vi "RIB Req - UDP Enable ROV A B TMS.vi"(0 "Limits File Path":path, 5 "Results File Path":path, 11 "error in":errorcluster) -> (4 "Results Data Array":string[][](array[string]), 15 "error out":errorcluster)   [LabVIEW 2024]
doc: "Template test"
uses:
  <vilib>/addons/_JKI Toolkits/State Machine/_JKI_lib_State_Machine.llb/Select State(s)_err__jki_lib_state_machine.vi
  <vilib>/addons/_JKI Toolkits/State Machine/_JKI_lib_State_Machine.llb/Select State(s)_bool__jki_lib_state_machine.vi
  <vilib>/addons/_JKI Toolkits/State Machine/_JKI_lib_State_Machine.llb/Periodic Trigger__ogtk__JKI-SM__jki_lib_state_machine.vi
  <userlib>/_OpenG.lib/file/file.llb/Strip Path Extension - String__ogtk.vi
  <vilib>/Utility/file.llb/Read Delimited Spreadsheet (string).vi
  <userlib>/_OpenG.lib/file/file.llb/openg_file.lvlib
  <userlib>/_OpenG.lib/appcontrol/appcontrol.llb/openg_application_control.lvlib
  <userlib>/_OpenG.lib/time/time.llb/openg_time.lvlib
  <vilib>/Utility/file.llb/Write Delimited Spreadsheet (string).vi
panel:
  in  "Connect":string
  in  "Connect Fail":string
  out "Timeout (Read States) 3":dbl(slide) scale=0.0..10.0
  out "Timeout (Read States)":dbl(slide) scale=0.0..15.0
  out "Timeout (Read States) 2":dbl(slide) scale=0.0..10.0
  out "ROV A Enabled":bool
  out "ROV B Enabled":bool
  out "TMS Enabled":bool
  in  "Read Normal Operation":string
  in  "Read Wait for Start":string
  in  "Read TMS":string
  in  "Read ROV B":string
  in  "Read ROV A":string
  out "Results Data 8":string[](array[string])
  out "Results Data 7":string[](array[string])
  out "Results Data 6":string[](array[string])
  in  "5A Test":bool
  in  "task out":refnum<k21>
  in  "UDP Read":string
  in  "connection ID":refnum<k16>
  in  "Exit":bool
  # "Enable ROV A, ROV B + TMS  Test"
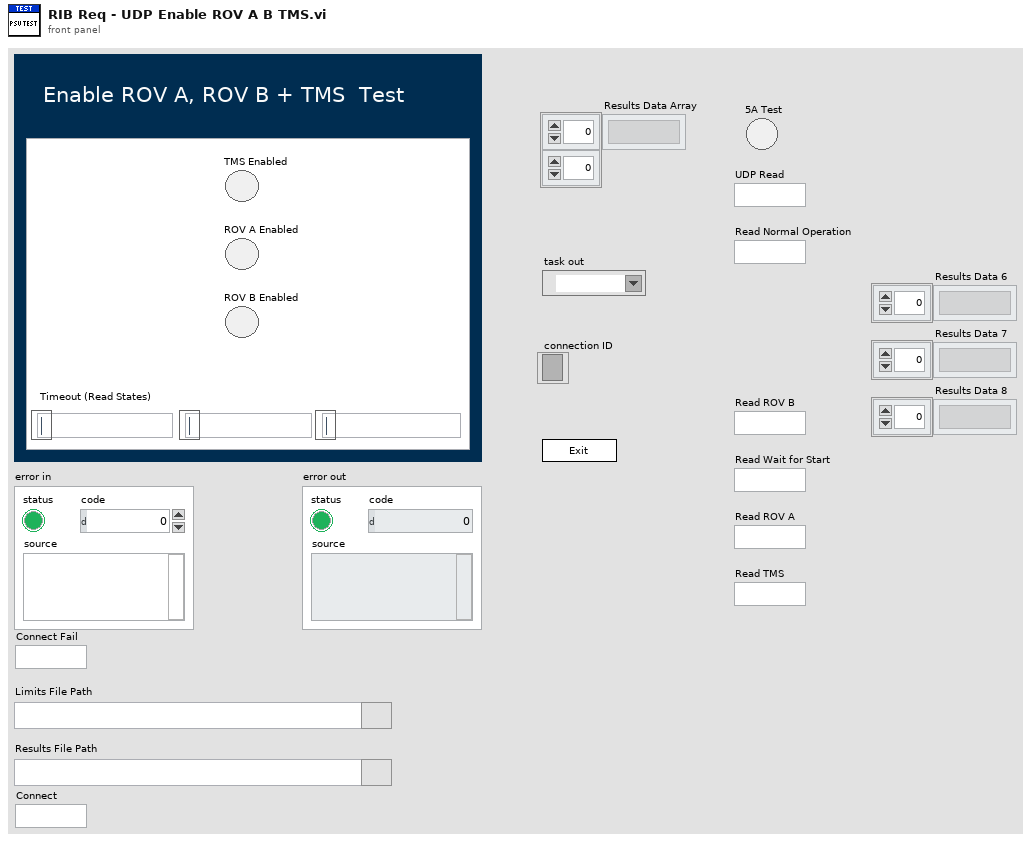
[diagram p1: front panel]
types:
  T1 = enum32{"Invalid", "Standard", "Closed", "Hidden", "Minimized", "Maximized"}
  T2 = enum32{"invalid app kind", "Development System", "Run Time System", "Student Edition", "Embedded LabVIEW", "Evaluation", "Custom"}
  T3 = typedef "FGV - Enum" = enum16{"Cleanup", "Get Data", "Open UDP", "Initialise DAQ", "Initialise I2C"}
  T4 = enum16{"Start Timer", "Get Time", "Pause", "Unpause"}
  T5 = cluster{"Core":cluster{"Current VI Reference":refnum<vi>, "Close Panel on Exit?":bool}, "Limits File Path":path, "Test Limits":string[][], "Results Data Array":string[][], "Results File Path":path, "UDP Read":string, "connection ID":refnum<k16>, "task out":refnum<k21>, "5A Test":bool, "Connect Fail":string, "Connect":string, "Read ROV A":string, "Read ROV B":string, "Read TMS":string, "Read Wait for Start":string, "Read Normal Operation":string}
  T6 = cluster{"Current VI Reference":refnum<vi>, "Close Panel on Exit?":bool}
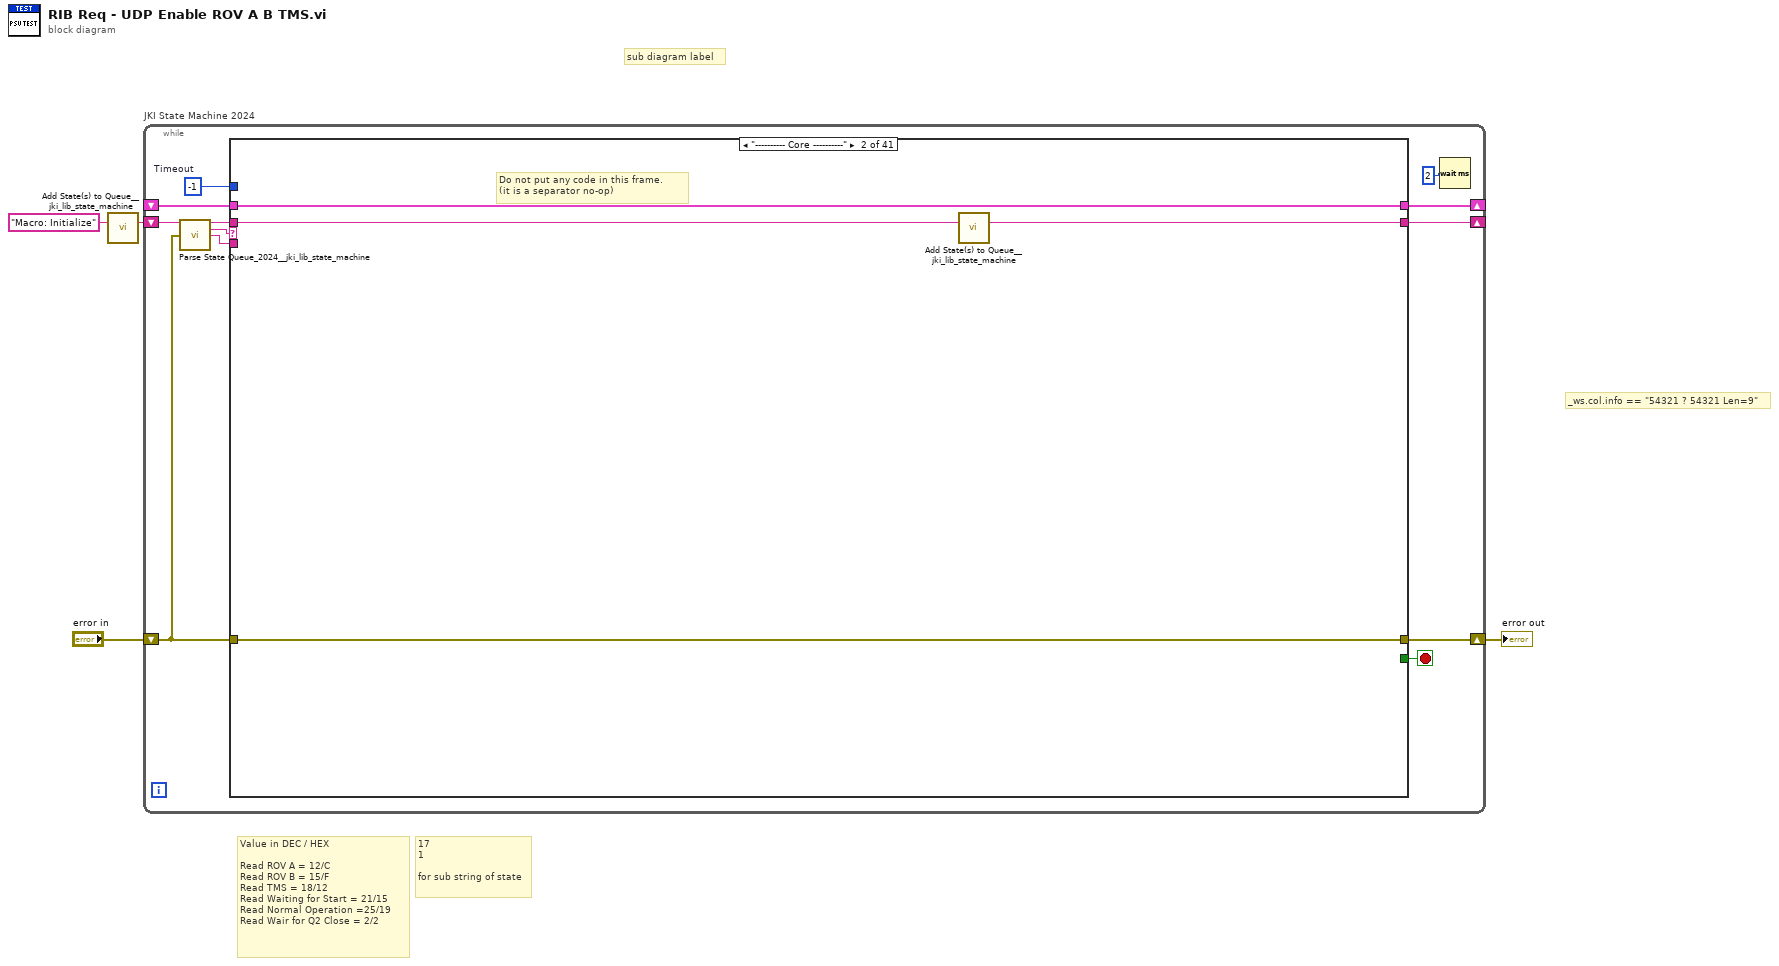
[diagram p0: block diagram]
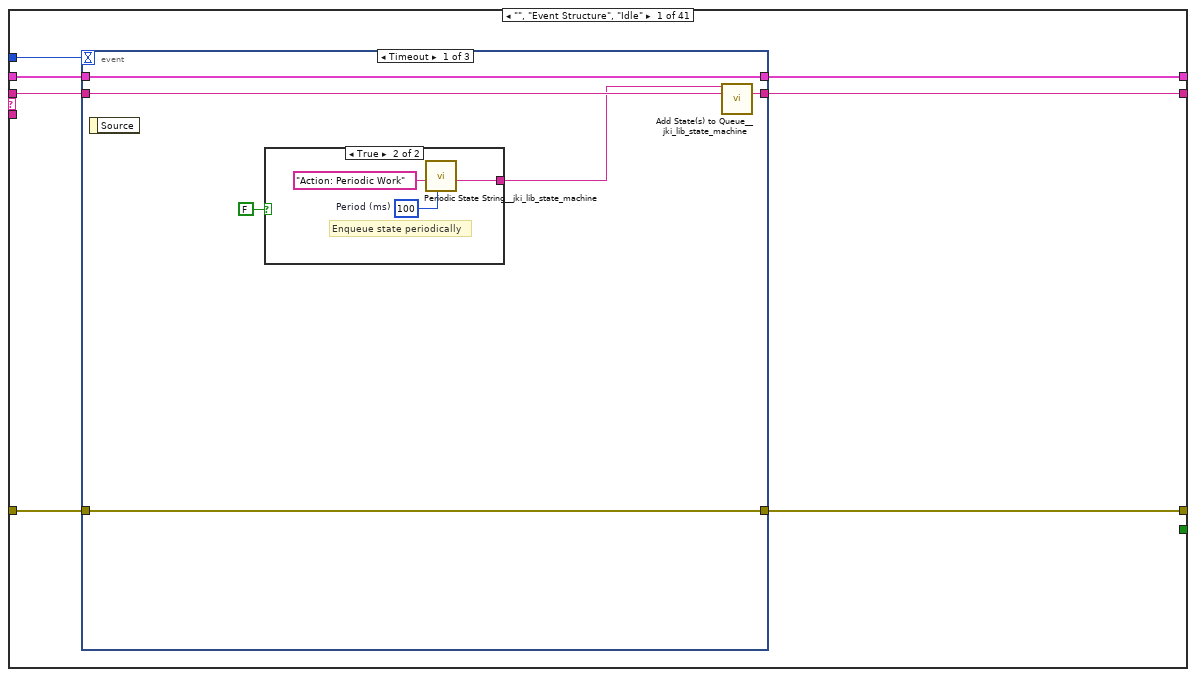
[diagram p2: hidden frame]
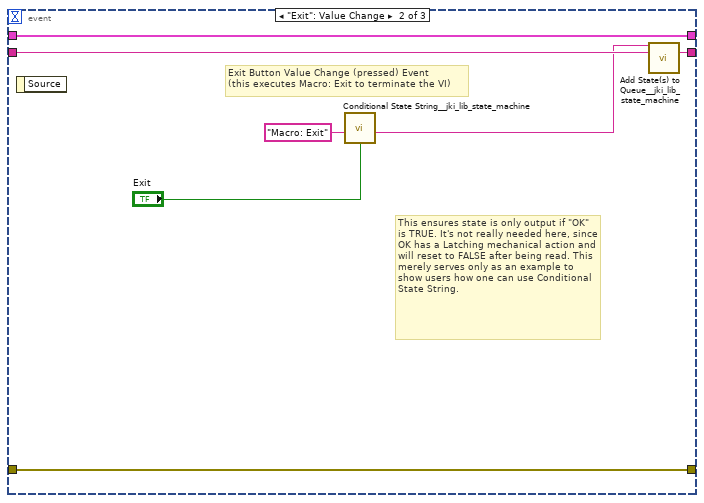
[diagram p4: hidden frame]
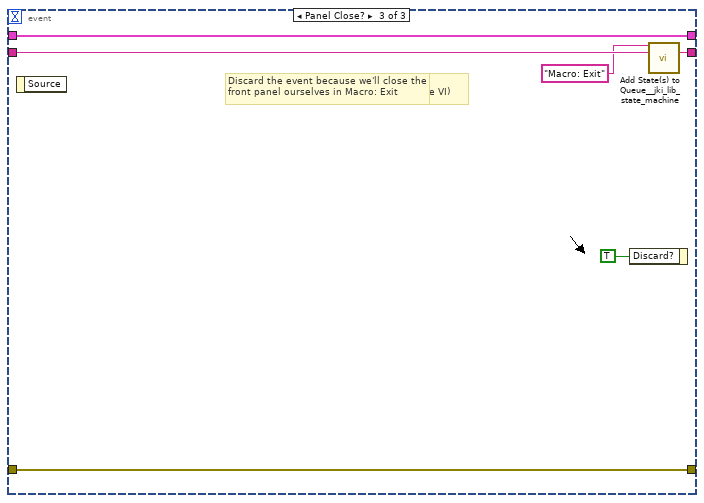
[diagram p5: hidden frame]
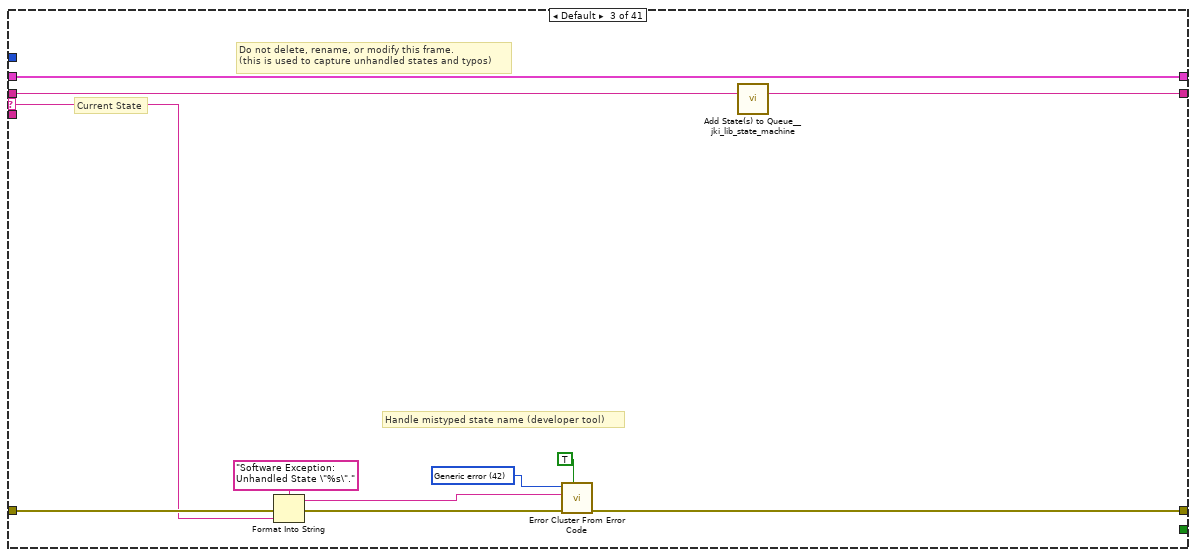
[diagram p6: hidden frame]
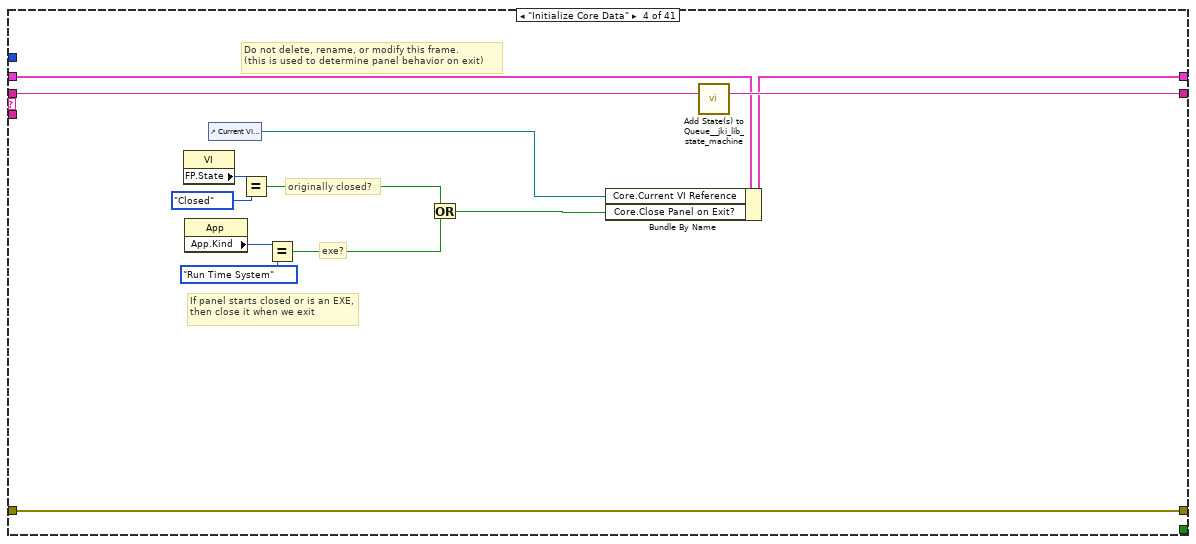
[diagram p7: hidden frame]
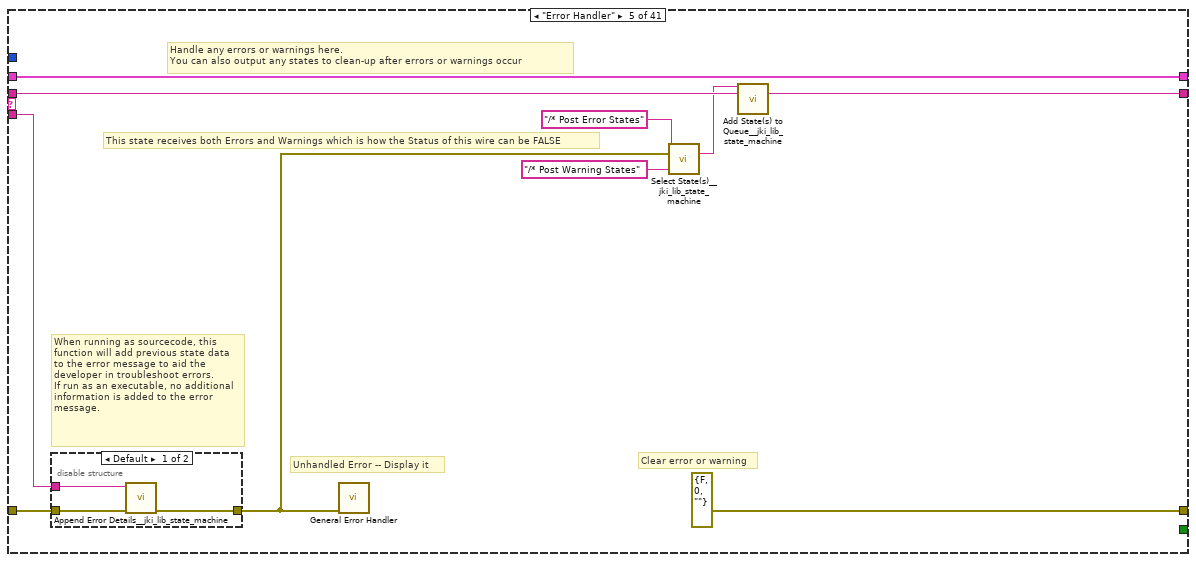
[diagram p8: hidden frame]
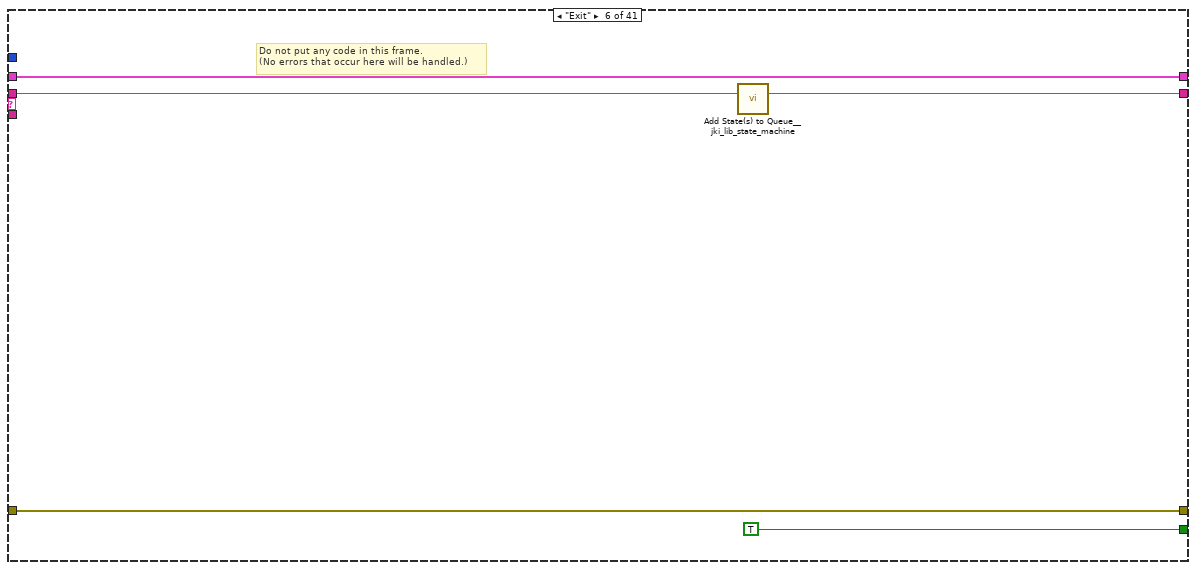
[diagram p10: hidden frame]
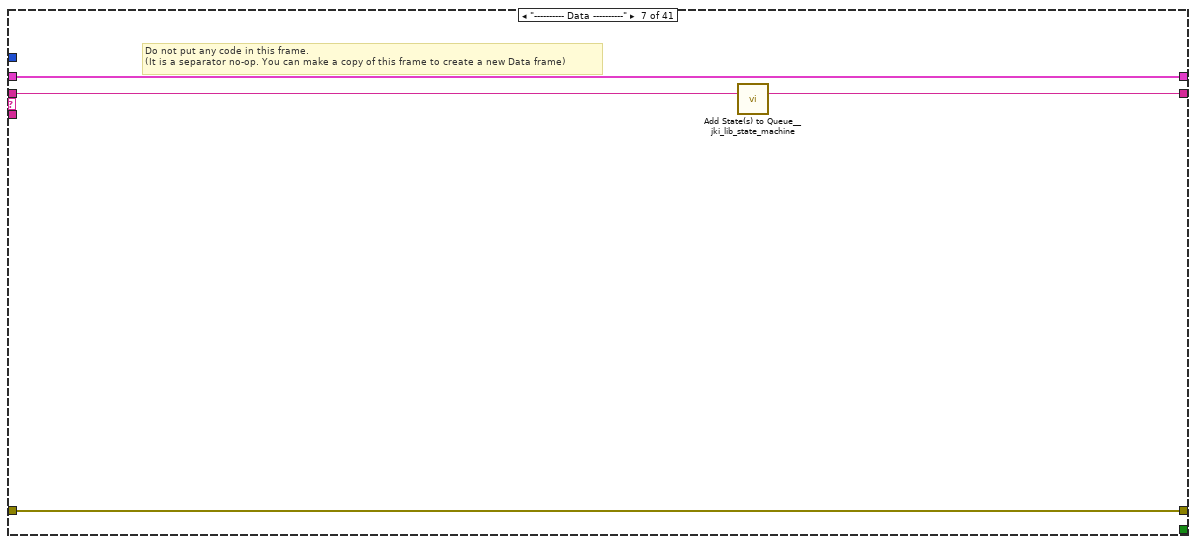
[diagram p11: hidden frame]
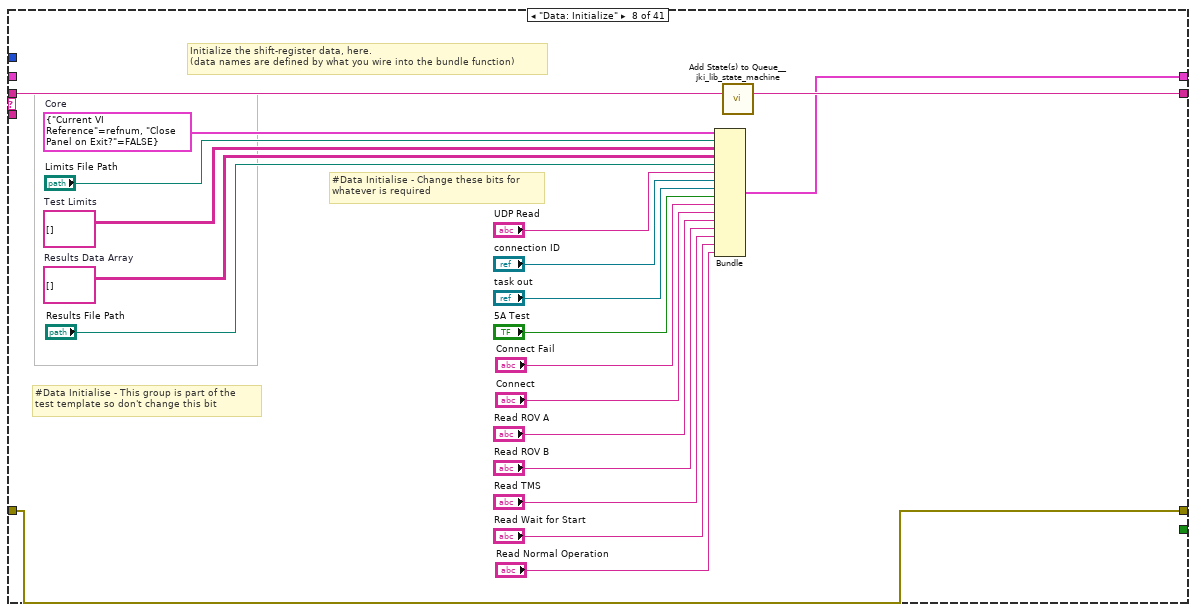
[diagram p12: hidden frame]
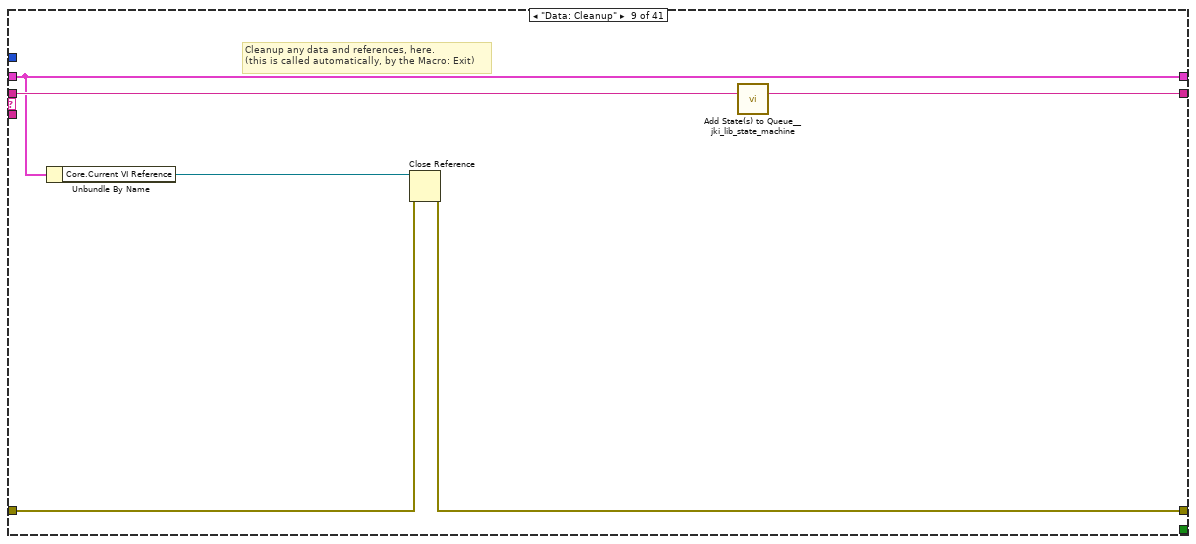
[diagram p13: hidden frame]
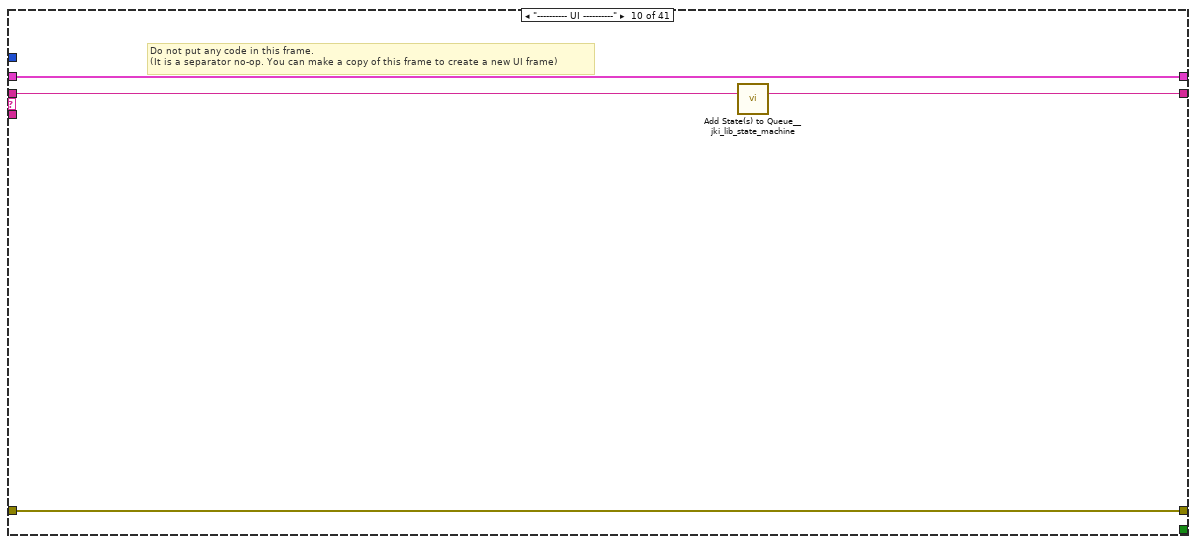
[diagram p14: hidden frame]
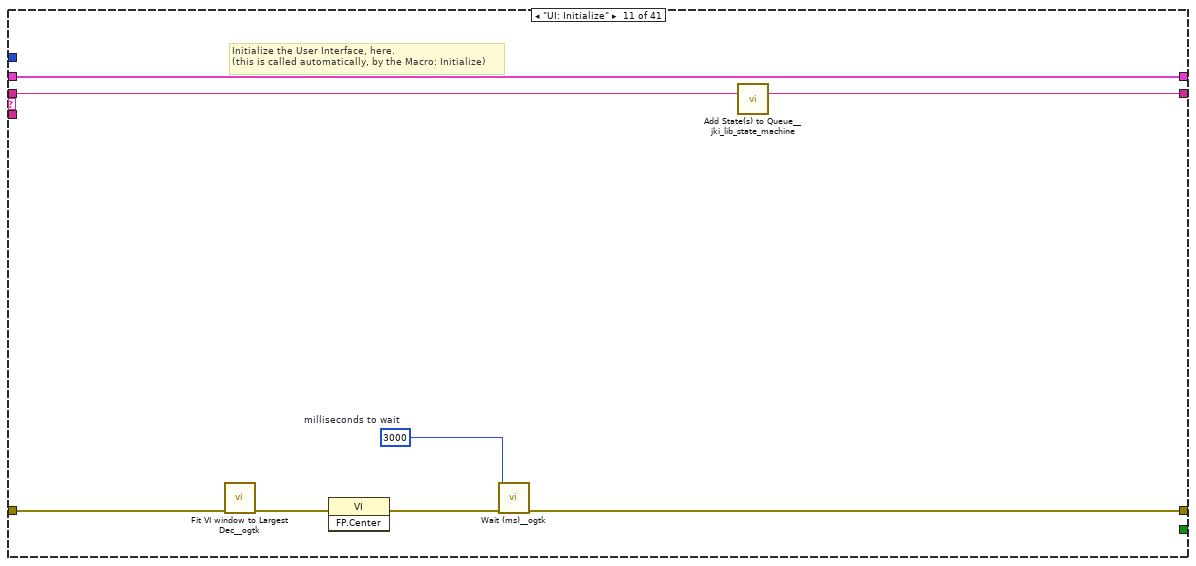
[diagram p15: hidden frame]
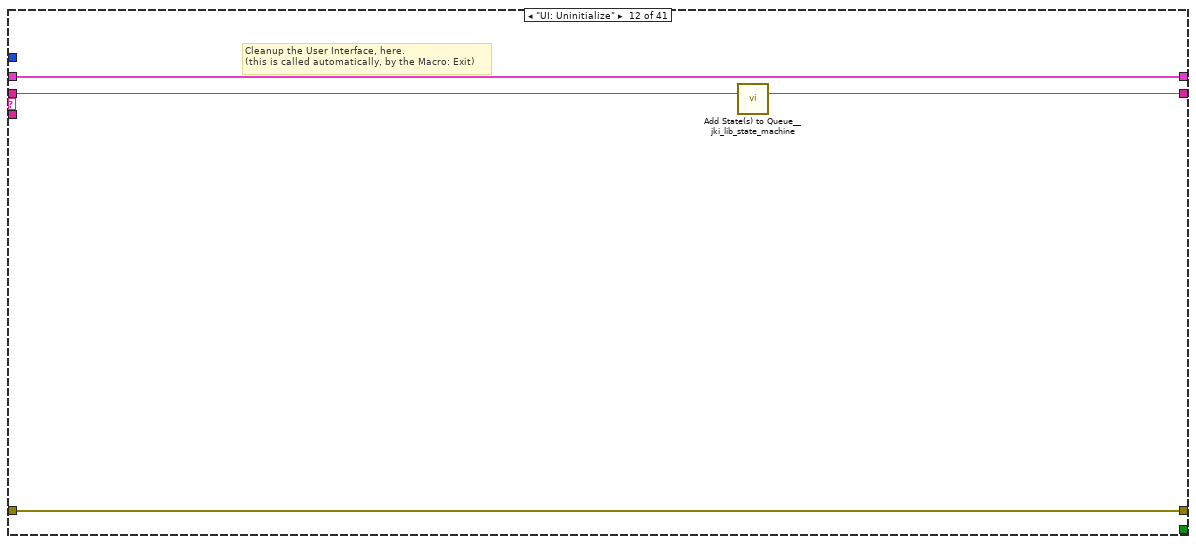
[diagram p16: hidden frame]
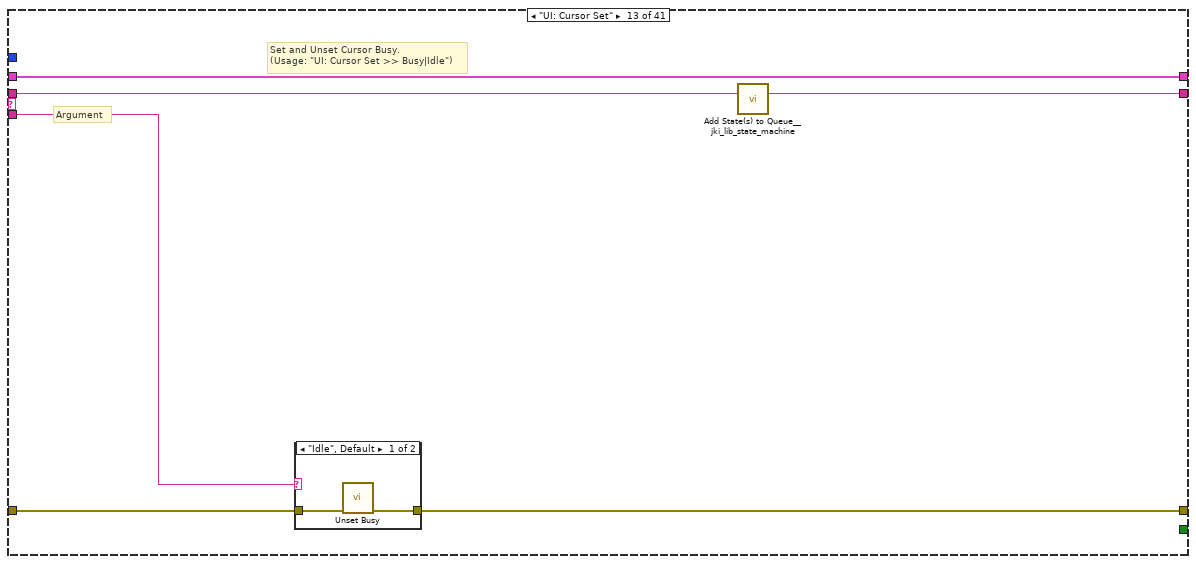
[diagram p17: hidden frame]
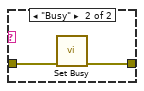
[diagram p18: hidden frame]
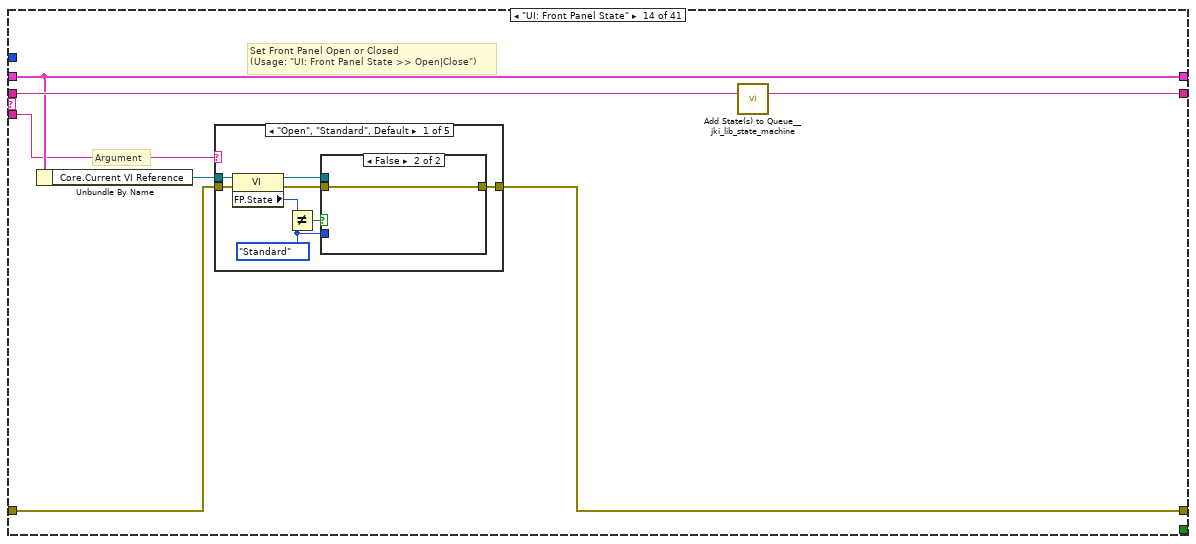
[diagram p19: hidden frame]
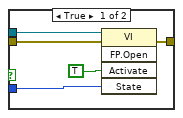
[diagram p20: hidden frame]
diagram:
  # "17\n1\n\nfor sub string of state"
  # "Value in DEC / HEX\n\nRead ROV A = 12/C\nRead ROV B = 15/F\nRead TMS = 18/12\nRead Waiting for Start = 21/15\nRead Normal Operation =25/19 \nRead Wair for Q2 Close = 2/2"
  # "_ws.col.info == \"54321 ? 54321 Len=9\""
  # "sub diagram label"
  n1 = call <vilib>:"Add State(s) to Queue__jki_lib_state_machine.vi"("State(s) in (\"\")"="Macro: Initialize") -> ("States Out"=w4:string)  [unwired: 14 in]
  n2 = while "JKI State Machine 2024" {
    shift-right: [w9] -> _
    shift-left: _ -> [w8]
    shift-right: [w12] -> w1
    shift-left: "error in" -> [w6]
    shift-right: [w11] -> _
    shift-left: w4 -> [w13]
    stop <- w10 stop-if-true
    w7 = -1  # Timeout
    n3 = call <vilib>:"Parse State Queue_2024__jki_lib_state_machine.vi"("State Queue"=w13, "Error In (no error)"=w6) -> ("Remaining States"=w15:string, "Current State"=w16:string, "Arguments"=w14:string)  [unwired: 11 in]
    n4 = case shown="\"---------- Core ----------\"" w16 {
      selector: w16 -> [_ _ w50 _ _ _ _ _ _ _ _ _ _ _ _ _ _ _ _ _ _ _ _ _ _ _ _ _ _ _ _ _ _ _ _ _ _ _ _ _ _]
      tunnel: w15 -> [w23 w49 w54 w73 w83 w92 w96 w116 w122 w126 w134 w138 w144 w155 w224 w229 w234 w239 w244 w249 w258 w262 w275 w292 w305 w318 w322 w331 w335 w343 w387 w408 w418 w442 w454 w464 w488 w500 w510 w534 w546]
      tunnel: w14 -> [_ _ _ _ w78 _ _ _ _ _ _ _ w139 w149 _ _ _ _ _ _ _ _ _ _ _ _ _ _ _ _ _ _ _ _ _ _ _ _ _ _ _]
      tunnel: w8 -> [w21 w46 w52 w66 w80 w90 w93 _ w117 w123 w132 w136 w142 w151 w221 w226 w231 w236 w241 w246 w256 w259 w265 w284 w297 w310 w319 w327 w332 w341 w351 w405 w416 w428 w452 w462 w471 w498 w508 w517 w544]
      tunnel: [w20 w47 w56 w70 errorcluster {"status"=FALSE, "code"=0, "source"=""} ("error out") w89 w94 w113 w118 w124 w130 w135 w140 w152 w222 w227 w232 w237 w242 w247 w253 w260 w271 w289 w302 w315 w320 w329 w333 w338 w346 w389 w409 w426 w449 w455 w467 w495 w501 w513 w541] -> w12
      tunnel: w6 -> [w17 w47 w55 w70 w79 w89 w94 w113 w119 w124 w131 w135 w141 w153 w222 w227 w232 w237 w242 w247 w253 w260 w270 w288 w301 w314 w320 w328 w333 w337 w354 w394 w414 w425 w450 w460 w466 w496 w506 w512 w542]
      tunnel: [w22 w48 w53 w72 w82 w91 w95 w115 w121 w125 w133 w137 w143 w154 w223 w228 w233 w238 w243 w248 w257 w261 w274 w291 w304 w317 w321 w330 w334 w342 w386 w407 w417 w441 w453 w463 w487 w499 w509 w533 w545] -> w11
      tunnel: [_ _ _ _ _ TRUE _ _ _ _ _ _ _ _ _ _ _ _ _ _ _ _ _ _ _ _ _ _ _ _ _ _ _ _ _ _ _ _ _ _ _] -> w10
      tunnel: [w19 w46 w52 w71 w80 w90 w93 w114 w117 w123 w132 w136 w142 w151 w221 w226 w231 w236 w241 w246 w256 w259 w264 w283 w296 w309 w319 w327 w332 w340 w385 w406 w416 w427 w452 w462 w470 w498 w508 w516 w544] -> w9
      tunnel: w7 -> [w18 _ _ _ _ _ _ _ _ _ _ _ _ _ _ _ _ _ _ _ _ _ _ _ _ _ _ _ _ _ _ _ _ _ _ _ _ _ _ _ _]
      frame "", "Event Structure", "Idle" {
        n5 = event shown="[0] Timeout" {
          selector: _ -> [_ _ _]
          dyn-events: _ -> [_ _ _]
          timeout: w18 -> [_ _ _]
          tunnel: w23 -> [w29 w39 w45]
          tunnel: [w28 w38 w44] -> w22
          tunnel: w21 -> [w26 w36 w42]
          tunnel: [w27 w37 w43] -> w20
          tunnel: w17 -> [w27 w37 w43]
          tunnel: [w26 w36 w42] -> w19
          event Timeout {
            n6 = event-data() -> ()  [unwired: 1 in, 1 out]
            n7 = case shown="True" FALSE {
              tunnel: [_ w32] -> w25
              frame False {
              }
              frame True {
                w30 = u32 100  # Period (ms)
                # "Enqueue state periodically"
                n8 = call <vilib>:"Periodic State String__jki_lib_state_machine.vi"("Period (ms)"=w30, "State"="Action: Periodic Work") -> ("State Out"=w32:string)  [unwired: 9 in]
              }
            }
            n9 = call <vilib>:"Add State(s) to Queue__jki_lib_state_machine.vi"("State(s) in Front (\"\")"=w25, "State(s) in (\"\")"=w29) -> ("States Out"=w28:string)  [unwired: 13 in]
          }
          event "Exit": Value Change {
            # "This ensures state is only output if \"OK\" is TRUE. It's not really needed here, since OK has a Latching mechanical action and will reset to FALSE after being read. This merely serves only as an example to show users how one can use Conditional State String."
            # "Exit Button Value Change (pressed) Event\n(this executes Macro: Exit to terminate the VI)"
            n10 = event-data() -> ()  [unwired: 1 in, 1 out]
            n11 = call <vilib>:"Conditional State String__jki_lib_state_machine.vi"("Do State(s)?"="Exit", "State"="Macro: Exit") -> ("State Out"=w33:string)  [unwired: 7 in]
            n12 = call <vilib>:"Add State(s) to Queue__jki_lib_state_machine.vi"("State(s) in Front (\"\")"=w33, "State(s) in (\"\")"=w39) -> ("States Out"=w38:string)  [unwired: 13 in]
          }
          event Panel Close? {
            # "Discard the event because we'll close the front panel ourselves in Macro: Exit"
            # "Close Panel button (pressed) Event\n(this executes Macro: Exit to terminate the VI)"
            n13 = event-data() -> ()  [unwired: 1 in, 1 out]
            n14 = event-data("Discard?"=TRUE) -> ()  [unwired: 1 in, 1 out]
            n15 = call <vilib>:"Add State(s) to Queue__jki_lib_state_machine.vi"("State(s) in Front (\"\")"="Macro: Exit", "State(s) in (\"\")"=w45) -> ("States Out"=w44:string)  [unwired: 13 in]
          }
        }
      }
      frame "---------- Core ----------" {
        # "Do not put any code in this frame.\n(it is a separator no-op)"
        n16 = call <vilib>:"Add State(s) to Queue__jki_lib_state_machine.vi"("State(s) in (\"\")"=w49) -> ("States Out"=w48:string)  [unwired: 14 in]
      }
      frame Default {
        w59 = 42 items=["No error", "Argument error", "Memory is full", "Out of zone", "End of file", "File already open", "Generic file I/O error", "File not found", "File permission error", "Disk is full", "Duplicate path", "Too many files open", "System feature not enabled", "Resource file not found", "Cannot add resource", "Resource not found", "Image not found", "Image memory error", "Pen does not exist", "Config type invalid", "Config token not found", "Config parse error", "Config memory error", "Bad external code format", "Bad external code offset", "External code not present", "Null window", "Destroy window error", "Null menu", "Print aborted", "Bad print record", "Print driver error", "Windows error during printing", "Memory error during printing", "Print dialog error", "Generic print error", "Invalid device refnum", "Device not found", "Device parameter error", "Device unit error", "Cannot open device", "Device call aborted", "Generic error", "Cancelled by user", "Object ID too low", "Object ID too high", "Object not in heap", "Unknown heap", "Unknown object (invalid DefProc)", "Unknown object (DefProc not in table)", "Message out of range", "Invalid (null) method", "Unknown message", "Manager call not supported", "Bad address", "Network operation in progress", "Network operation timed out", "Connection is busy", "Network attribute not supported", "Network error", "Address in use", "System out of memory", "Connection aborted", "Connection refused", "Not connected", "Already connected", "Connection closed", "Initialization error (interapplication manager)", "Bad occurrence", "Wait on unbound occurrence handler", "Occurrence queue overflow", "Datalog type conflict", "Unused", "Unrecognized type (interapplication manager)", "Memory corrupt", "Failed to make temporary DLL", "Old CIN version", "Drag socket not found", "Failed to load drop-object", "Failed to register OLE object", "Failed to release OLE object", "Format specifier type mismatch", "Unknown format specifier", "Too few format specifiers", "Too many format specifiers", "Scan failed", "Newer CIN version", "Error converting to variant", "Runtime menu error", "Password tampered", "Variant attribute not found", "Incompatible variant data type", "Event data is not available", "Event Store is not present", "Occurrence is not found", "Event Queue is not created", "Event info is not available", "Refnum passed is NULL", "Error retrieving Class GUID", "Error retrieving CoClass GUID", "Error retrieving TypeLib GUID.", "Bad built application magic bytes.", "Specific driver is different from the specific driver associated with the Logical Name.", "There is no session opened to the class driver.", "Max Error", "MAX - Error with config objects", "MAX - Error loading configuration", "MAX - Group not supported"]
        # "Current State"
        # "Do not delete, rename, or modify this frame.\n(this is used to capture unhandled states and typos)"
        # "Handle mistyped state name (developer tool)"
        n17 = Format Into String(format string="Software Exception: Unhandled State \"%s\"." ("message"), error in=w55, w50) -> (resulting string=w58:string, error out=w57:errorcluster)  [unwired: 1 in]
        n18 = call <vilib>:"Error Cluster From Error Code.vi"("show call chain? (False)"=TRUE, "error in (no error)"=w57, "error message (\"\")"=w58, "error code (0)"=w59) -> ("error out"=w56:errorcluster)  [unwired: 5 in]
        n19 = call <vilib>:"Add State(s) to Queue__jki_lib_state_machine.vi"("State(s) in (\"\")"=w54) -> ("States Out"=w53:string)  [unwired: 14 in]
      }
      frame "Initialize Core Data" {
        # "Do not delete, rename, or modify this frame.\n(this is used to determine panel behavior on exit)"
        # "originally closed?"
        # "exe?"
        # "If panel starts closed or is an EXE, then close it when we exit"
        n20 = property class="VI"() -> ("FP.State"=w63:T1)  [unwired: 2 in, 2 out]
        n21 = property class="App"() -> ("App.Kind"=w69:T2)  [unwired: 2 in, 2 out]
        n22 = control-ref of="Current VI Reference"() -> (w64:refnum<vi>)
        n23 = Equal?(x=w63, y=T1."Closed" ("Front Panel Window:State")) -> (x = y?=w61:bool)
        n24 = Equal?(x=w69, y=T2."Run Time System" ("Application:Kind")) -> (x = y?=w67:bool)
        n25 = Or(x=w61, y=w67) -> (x .or. y?=w65:bool)
        n26 = Bundle By Name(cluster=w66, "Core.Current VI Reference"=w64, "Core.Close Panel on Exit?"=w65) -> (w71:T5)
        n27 = call <vilib>:"Add State(s) to Queue__jki_lib_state_machine.vi"("State(s) in (\"\")"=w73) -> ("States Out"=w72:string)  [unwired: 14 in]
      }
      frame "Error Handler" {
        # "When running as sourcecode, this function will add previous state data to the error message to aid the developer in troubleshoot errors.\nIf run as an executable, no additional information is added to the error message."
        # "This state receives both Errors and Warnings which is how the Status of this wire can be FALSE"
        # "Unhandled Error -- Display it"
        # "Handle any errors or warnings here.\nYou can also output any states to clean-up after errors or warnings occur"
        # "Clear error or warning"
        n28 = disable-structure shown="Default" {
          disable-tunnel: w79 -> [w86 w87]
          disable-tunnel: w78 -> [w85 _]
          disable-tunnel: [w84 w87] -> w77
          frame condition #0 (active) {
            n29 = call <vilib>:"Append Error Details__jki_lib_state_machine.vi"("error in (no error)"=w86, "Previous State and Argument(s)"=w85) -> ("error out"=w84:errorcluster)  [unwired: 9 in]
          }
          frame condition #1 {
          }
        }
        n30 = call <vilib>:"General Error Handler.vi"("error in (no error)"=w77) -> ()  [unwired: 10 in, 5 out]
        n31 = call-poly <vilib>:"Select State(s)__jki_lib_state_machine.vi"("State(s) if True (\"\")"="/* Post Error States", "Select"=w77, "State(s) if False (\"\")"="/* Post Warning States") -> ("States Out"=w75:string)  [unwired: 12 in]
        n32 = call <vilib>:"Add State(s) to Queue__jki_lib_state_machine.vi"("State(s) in Front (\"\")"=w75, "State(s) in (\"\")"=w83) -> ("States Out"=w82:string)  [unwired: 13 in]
      }
      frame "Exit" {
        # "Do not put any code in this frame.\n(No errors that occur here will be handled.)"
        n33 = call <vilib>:"Add State(s) to Queue__jki_lib_state_machine.vi"("State(s) in (\"\")"=w92) -> ("States Out"=w91:string)  [unwired: 14 in]
      }
      frame "---------- Data ----------" {
        # "Do not put any code in this frame.\n(It is a separator no-op. You can make a copy of this frame to create a new Data frame)"
        n34 = call <vilib>:"Add State(s) to Queue__jki_lib_state_machine.vi"("State(s) in (\"\")"=w96) -> ("States Out"=w95:string)  [unwired: 14 in]
      }
      frame "Data: Initialize" {
        w109 = string[][] []  # Results Data Array
        w110 = string[][] []  # Test Limits
        w112 = T6 {"Current VI Reference"=refnum, "Close Panel on Exit?"=FALSE}  # Core
        # "#Data Initialise - Change these bits for\nwhatever is required"
        # "#Data Initialise - This group is part of the\ntest template so don't change this bit"
        # "Initialize the shift-register data, here.\n(data names are defined by what you wire into the bundle function)"
        n35 = Bundle("Core"=w112, "Limits File Path"="Limits File Path", "Test Limits"=w110, "Results Data Array"=w109, "Results File Path"="Results File Path", "UDP Read"="UDP Read", "connection ID"="connection ID", "task out"="task out", "5A Test"="5A Test", "Connect Fail"="Connect Fail", "Connect"="Connect", "Read ROV A"="Read ROV A", "Read ROV B"="Read ROV B", "Read TMS"="Read TMS", "Read Wait for Start"="Read Wait for Start", "Read Normal Operation"="Read Normal Operation") -> (w114:T5)  [unwired: 1 in]
        n36 = call <vilib>:"Add State(s) to Queue__jki_lib_state_machine.vi"("State(s) in (\"\")"=w116) -> ("States Out"=w115:string)  [unwired: 14 in]
      }
      frame "Data: Cleanup" {
        # "Cleanup any data and references, here.\n(this is called automatically, by the Macro: Exit)"
        n37 = Unbundle By Name(w117) -> ("Core.Current VI Reference"=w120:refnum<vi>)
        n38 = Close Reference(reference=w120, error in (no error)=w119) -> (error out=w118:errorcluster)
        n39 = call <vilib>:"Add State(s) to Queue__jki_lib_state_machine.vi"("State(s) in (\"\")"=w122) -> ("States Out"=w121:string)  [unwired: 14 in]
      }
      frame "---------- UI ----------" {
        # "Do not put any code in this frame.\n(It is a separator no-op. You can make a copy of this frame to create a new UI frame)"
        n40 = call <vilib>:"Add State(s) to Queue__jki_lib_state_machine.vi"("State(s) in (\"\")"=w126) -> ("States Out"=w125:string)  [unwired: 14 in]
      }
      frame "UI: Initialize" {
        w129 = u32 3000  # milliseconds to wait
        # "Initialize the User Interface, here.\n(this is called automatically, by the Macro: Initialize)"
        n41 = call <userlib>:"Fit VI window to Largest Dec__ogtk.vi"("error in (no error)"=w131) -> ("error out"=w127:errorcluster)  [unwired: 5 in, 1 out]
        n42 = invoke class="VI" method="FP.Center"(error in=w127) -> (error out=w128:errorcluster)  [unwired: 2 in, 2 out]
        n43 = call <userlib>:"Wait (ms)__ogtk.vi"("error in (no error)"=w128, "milliseconds to wait"=w129) -> ("error out"=w130:errorcluster)  [unwired: 8 in, 1 out]
        n44 = call <vilib>:"Add State(s) to Queue__jki_lib_state_machine.vi"("State(s) in (\"\")"=w134) -> ("States Out"=w133:string)  [unwired: 14 in]
      }
      frame "UI: Uninitialize" {
        # "Cleanup the User Interface, here.\n(this is called automatically, by the Macro: Exit)"
        n45 = call <vilib>:"Add State(s) to Queue__jki_lib_state_machine.vi"("State(s) in (\"\")"=w138) -> ("States Out"=w137:string)  [unwired: 14 in]
      }
      frame "UI: Cursor Set" {
        # "Argument"
        # "Set and Unset Cursor Busy.\n(Usage: \"UI: Cursor Set >> Busy|Idle\")"
        n46 = case shown="\"Idle\", Default" w139 {
          tunnel: w141 -> [w146 w148]
          tunnel: [w145 w147] -> w140
          frame "Idle", Default {
            n47 = call <vilib>:"Unset Busy.vi"("error in (no error)"=w146) -> ("error out"=w145:errorcluster)  [unwired: 10 in]
          }
          frame "Busy" {
            n48 = call <vilib>:"Set Busy.vi"("error in (no error)"=w148) -> ("error out"=w147:errorcluster)  [unwired: 9 in, 1 out]
          }
        }
        n49 = call <vilib>:"Add State(s) to Queue__jki_lib_state_machine.vi"("State(s) in (\"\")"=w144) -> ("States Out"=w143:string)  [unwired: 14 in]
      }
      frame "UI: Front Panel State" {
        # "Argument"
        # "Set Front Panel Open or Closed\n(Usage: \"UI: Front Panel State >> Open|Close\")"
        n50 = Unbundle By Name(w151) -> ("Core.Current VI Reference"=w150:refnum<vi>)
        n51 = case shown="\"Open\", \"Standard\", Default" w149 {
          tunnel: w153 -> [w161 w176 w187 w200 w213]
          tunnel: [w163 w177 w189 w202 w215] -> w152
          tunnel: w150 -> [w162 w174 w188 w201 w214]
          frame "Open", "Standard", Default {
            w156 = T1."Standard" ("State")
            n52 = property class="VI"(reference=w162, error in=w161) -> (reference out=w159:refnum<vi>, error out=w160:errorcluster, "FP.State"=w158:T1)
            n53 = Not Equal?(x=w158, y=w156) -> (x != y?=w157:bool)
            n54 = case shown="False" w157 {
              tunnel: [w167 w169] -> w163
              tunnel: w160 -> [w166 w169]
              tunnel: w159 -> [w165 _]
              tunnel: w156 -> [w164 _]
              frame True {
                n55 = invoke class="VI" method="FP.Open"(reference=w165, error in=w166, "Activate"=TRUE, "State"=w164) -> (error out=w167:errorcluster)  [unwired: 1 in, 4 out]
              }
              frame False {
              }
            }
          }
          frame "Close", "Closed" {
            n56 = property class="VI"(reference=w174, error in=w176) -> (reference out=w173:refnum<vi>, error out=w175:errorcluster, "FP.State"=w171:T1)
            n57 = Not Equal?(x=w171, y=T1."Closed" ("Front Panel Window:State")) -> (x != y?=w170:bool)
            n58 = case shown="True" w170 {
              tunnel: [w178 w181] -> w177
              tunnel: w175 -> [w178 w180]
              tunnel: w173 -> [_ w179]
              frame False {
              }
              frame True {
                n59 = invoke class="VI" method="FP.Close"(reference=w179, error in=w180) -> (error out=w181:errorcluster)  [unwired: 1 in, 2 out]
              }
            }
          }
          frame "Hidden", "Hide" {
            w182 = T1."Hidden" ("State")
            n60 = property class="VI"(reference=w188, error in=w187) -> (reference out=w185:refnum<vi>, error out=w186:errorcluster, "FP.State"=w184:T1)
            n61 = Not Equal?(x=w184, y=w182) -> (x != y?=w183:bool)
            n62 = case shown="True" w183 {
              tunnel: [w193 w194] -> w189
              tunnel: w186 -> [w192 w194]
              tunnel: w185 -> [w191 _]
              tunnel: w182 -> [w190 _]
              frame True {
                n63 = invoke class="VI" method="FP.Open"(reference=w191, error in=w192, "State"=w190) -> (error out=w193:errorcluster)  [unwired: 2 in, 4 out]
              }
              frame False {
              }
            }
          }
          frame "Minimize", "Minimized" {
            w195 = T1."Minimized" ("State")
            n64 = property class="VI"(reference=w201, error in=w200) -> (reference out=w198:refnum<vi>, error out=w199:errorcluster, "FP.State"=w197:T1)
            n65 = Not Equal?(x=w197, y=w195) -> (x != y?=w196:bool)
            n66 = case shown="True" w196 {
              tunnel: [w206 w207] -> w202
              tunnel: w199 -> [w205 w207]
              tunnel: w198 -> [w204 _]
              tunnel: w195 -> [w203 _]
              frame True {
                n67 = invoke class="VI" method="FP.Open"(reference=w204, error in=w205, "State"=w203) -> (error out=w206:errorcluster)  [unwired: 2 in, 4 out]
              }
              frame False {
              }
            }
          }
          frame "Maximize", "Maximized" {
            w208 = T1."Maximized" ("State")
            n68 = property class="VI"(reference=w214, error in=w213) -> (reference out=w211:refnum<vi>, error out=w212:errorcluster, "FP.State"=w210:T1)
            n69 = Not Equal?(x=w210, y=w208) -> (x != y?=w209:bool)
            n70 = case shown="True" w209 {
              tunnel: [w219 w220] -> w215
              tunnel: w212 -> [w218 w220]
              tunnel: w211 -> [w217 _]
              tunnel: w208 -> [w216 _]
              frame True {
                n71 = invoke class="VI" method="FP.Open"(reference=w217, error in=w218, "State"=w216) -> (error out=w219:errorcluster)  [unwired: 2 in, 4 out]
              }
              frame False {
              }
            }
          }
        }
        n72 = call <vilib>:"Add State(s) to Queue__jki_lib_state_machine.vi"("State(s) in (\"\")"=w155) -> ("States Out"=w154:string)  [unwired: 14 in]
      }
      frame "---------- Macro ----------" {
        # "Do not put any code in this frame.\n(It is a separator no-op. You can make a copy of this frame to create a new Macro frame)"
        n73 = call <vilib>:"Add State(s) to Queue__jki_lib_state_machine.vi"("State(s) in (\"\")"=w224) -> ("States Out"=w223:string)  [unwired: 14 in]
      }
      frame "Macro: Initialize" {
        # "Initialization Macro\n(This is called once, when the VI starts)"
        n74 = call <vilib>:"Add State(s) to Queue__jki_lib_state_machine.vi"("State(s) in Front (\"\")"="Data: Initialize\nInitialize Core Data\nUI: Initialize\nUI: Front Panel State >> Open\nMacro: Test", "State(s) in (\"\")"=w229) -> ("States Out"=w228:string)  [unwired: 13 in]
      }
      frame "Macro: Test" {
        # "#Test Macro - Add the sequence \nfor measurments and limits testing here"
        n75 = call <vilib>:"Add State(s) to Queue__jki_lib_state_machine.vi"("State(s) in Front (\"\")"="Limits Test: Read Limits File\nEnable States: UDP Open\nEnable States: Enable ROV A, ROV B and TMS\nEnable States: Set Command\nEnable States: Start Timer (ROV A)\nEnable States: Read ROV A State", "State(s) in (\"\")"=w234) -> ("States Out"=w233:string)  [unwired: 13 in]
      }
      frame "Macro: Test 2" {
        # "#Test Macro - Add the sequence \nfor measurments and limits testing here"
        n76 = call <vilib>:"Add State(s) to Queue__jki_lib_state_machine.vi"("State(s) in Front (\"\")"="Enable States: Start Timer (ROV B)\nEnable States: Read ROV B State", "State(s) in (\"\")"=w239) -> ("States Out"=w238:string)  [unwired: 13 in]
      }
      frame "Macro: Test 3" {
        # "#Test Macro - Add the sequence \nfor measurments and limits testing here"
        n77 = call <vilib>:"Add State(s) to Queue__jki_lib_state_machine.vi"("State(s) in Front (\"\")"="Enable States: Start Timer (TMS)\nEnable States: Read TMS State", "State(s) in (\"\")"=w244) -> ("States Out"=w243:string)  [unwired: 13 in]
      }
      frame "Macro: Limits" {
        # "Do not put any code in this frame.\n(It is a separator no-op. You can make a copy of this frame to create a new Macro frame)"
        n78 = call <vilib>:"Add State(s) to Queue__jki_lib_state_machine.vi"("State(s) in Front (\"\")"="Limits Test: Read ROV A Test\nLimits Test: Read ROV B Test\nLimits Test: Read TMS Test\nResults Data: Write Results Data\nMacro: Exit", "State(s) in (\"\")"=w249) -> ("States Out"=w248:string)  [unwired: 13 in]
      }
      frame "Macro: Exit" {
        # "Exit Macro\n(This is called once, when the VI exits)"
        n79 = Unbundle By Name(w256) -> ("Core.Close Panel on Exit?"=w251:bool)
        n80 = call <vilib>:"Conditional State String__jki_lib_state_machine.vi"("Do State(s)?"=w251, "State"="UI: Front Panel State >> Close") -> ("State Out"=w250:string)  [unwired: 7 in]
        n81 = call <vilib>:"Add State(s) to Queue__jki_lib_state_machine.vi"("State(s) in (\"\")"=w250, "State(s) at Back (\"\")"="UI: Uninitialize\nData: Cleanup\nExit") -> ("States Out"=w254:string)  [unwired: 13 in]
        n82 = call <vilib>:"Add State(s) to Queue__jki_lib_state_machine.vi"("State(s) in Front (\"\")"=w254, "State(s) in (\"\")"=w258) -> ("States Out"=w257:string)  [unwired: 13 in]
      }
      frame "---------- Limits Test ----------" {
        # "Template Separator\n(You can make a copy of, or modify, this frame)"
        n83 = call <vilib>:"Add State(s) to Queue__jki_lib_state_machine.vi"("State(s) in (\"\")"=w262) -> ("States Out"=w261:string)  [unwired: 14 in]
      }
      frame "Limits Test: Read Limits File" {
        w268 = ","  # delimiter (\t)
        n84 = Unbundle By Name(w265) -> ("Limits File Path"=w269:path)
        n85 = Current VI's Path "Test Case Path"() -> (path=w273:path)
        n86 = call-poly <vilib>:"Read Delimited Spreadsheet.vi"("file path (dialog if empty)"=w269, "error in (no error)"=w270, "delimiter (\\t)"=w268) -> ("all rows"=w266:string[][], "error out"=w271:errorcluster)  [unwired: 7 in, 4 out]
        n87 = Strip Path(path=w273) -> (name=w272:string)  [unwired: 1 out]
        n88 = call-poly <userlib>:"Strip Path Extension__ogtk.vi"("path"=w272) -> ("root"=w267:string)  [unwired: 1 out]
        n89 = for {
          tunnel: w267 -> [w279]
          tunnel: w266 -> [w277] mode=indexing
          tunnel: [w277] -> w263 mode=indexing if=w276
          n90 = Index Array(array=w277) -> (element=w278:string)  [unwired: 1 in]
          n91 = Equal?(x=w279, y=w278) -> (x = y?=w276:bool)
        }
        n92 = Bundle By Name(cluster=w265, "Test Limits"=w263) -> (w264:T5)
        n93 = call <vilib>:"Add State(s) to Queue__jki_lib_state_machine.vi"("State(s) in (\"\")"=w275) -> ("States Out"=w274:string)  [unwired: 14 in]
      }
      frame "Limits Test: Read ROV A Test" {
        w285 = "Read ROV A Test"  # Sub Test Name
        # "UDP Read Test = if equal to F0 = pass else fail"
        # "#Limits Testing - Add the sub test name for\ntest included in limits file"
        n94 = Unbundle By Name(w284) -> ("Test Limits"=w286:string[][], "Read ROV A"=w290:string)
        n95 = Unbundle By Name(w284) -> ("Results Data Array"=w282:string[][])
        n96 = To Variant(anything=w290) -> (Variant=w287:variant)
        n97 = call "Process Results.vi"("error in (no error)"=w288, "Measurement"=w287, "Test Limits"=w286, "Sub Test Name"=w285) -> ("error out"=w289:errorcluster, "Results Data"=w280:string[])  [unwired: 6 in]
        "Results Data 6" <- w280
        n98 = Build Array (concatenate)(w282, w280) -> (w281:string[][])
        n99 = Bundle By Name(cluster=w284, "Results Data Array"=w281) -> (w283:T5)
        n100 = call <vilib>:"Add State(s) to Queue__jki_lib_state_machine.vi"("State(s) in (\"\")"=w292) -> ("States Out"=w291:string)  [unwired: 14 in]
      }
      frame "Limits Test: Read ROV B Test" {
        w298 = "Read ROV B Test"  # Sub Test Name
        # "UDP Read Test = if equal to F0 = pass else fail"
        # "#Limits Testing - Add the sub test name for\ntest included in limits file"
        n101 = Unbundle By Name(w297) -> ("Test Limits"=w299:string[][], "Read ROV B"=w303:string)
        n102 = Unbundle By Name(w297) -> ("Results Data Array"=w295:string[][])
        n103 = To Variant(anything=w303) -> (Variant=w300:variant)
        n104 = call "Process Results.vi"("error in (no error)"=w301, "Measurement"=w300, "Test Limits"=w299, "Sub Test Name"=w298) -> ("error out"=w302:errorcluster, "Results Data"=w293:string[])  [unwired: 6 in]
        "Results Data 7" <- w293
        n105 = Build Array (concatenate)(w295, w293) -> (w294:string[][])
        n106 = Bundle By Name(cluster=w297, "Results Data Array"=w294) -> (w296:T5)
        n107 = call <vilib>:"Add State(s) to Queue__jki_lib_state_machine.vi"("State(s) in (\"\")"=w305) -> ("States Out"=w304:string)  [unwired: 14 in]
      }
      frame "Limits Test: Read TMS Test" {
        w311 = "Read TMS Test"  # Sub Test Name
        # "UDP Read Test = if equal to F0 = pass else fail"
        # "#Limits Testing - Add the sub test name for\ntest included in limits file"
        n108 = Unbundle By Name(w310) -> ("Results Data Array"=w308:string[][])
        n109 = Unbundle By Name(w310) -> ("Test Limits"=w312:string[][], "Read TMS"=w316:string)
        n110 = To Variant(anything=w316) -> (Variant=w313:variant)
        n111 = call "Process Results.vi"("error in (no error)"=w314, "Measurement"=w313, "Test Limits"=w312, "Sub Test Name"=w311) -> ("error out"=w315:errorcluster, "Results Data"=w306:string[])  [unwired: 6 in]
        "Results Data 8" <- w306
        n112 = Build Array (concatenate)(w308, w306) -> (w307:string[][])
        n113 = Bundle By Name(cluster=w310, "Results Data Array"=w307) -> (w309:T5)
        n114 = call <vilib>:"Add State(s) to Queue__jki_lib_state_machine.vi"("State(s) in (\"\")"=w318) -> ("States Out"=w317:string)  [unwired: 14 in]
      }
      frame "---------- Results Data ----------" {
        # "Template Separator\n(You can make a copy of, or modify, this frame)"
        n115 = call <vilib>:"Add State(s) to Queue__jki_lib_state_machine.vi"("State(s) in (\"\")"=w322) -> ("States Out"=w321:string)  [unwired: 14 in]
      }
      frame "Results Data: Write Results Data" {
        w324 = ","  # delimiter (\t)
        w325 = TRUE  # append to file? (new file:F)
        n116 = Unbundle By Name(w327) -> ("Results File Path"=w326:path, "Results Data Array"=w323:string[][])
        "Results Data Array" <- w323
        n117 = call-poly <vilib>:"Write Delimited Spreadsheet.vi"("file path (dialog if empty)"=w326, "2D data"=w323, "append to file? (new file:F)"=w325, "error in (no error)"=w328, "delimiter (\\t)"=w324) -> ("error out"=w329:errorcluster)  [unwired: 9 in, 1 out]
        n118 = call <vilib>:"Add State(s) to Queue__jki_lib_state_machine.vi"("State(s) in (\"\")"=w331) -> ("States Out"=w330:string)  [unwired: 14 in]
      }
      frame "---------- Enable States ----------" {
        # "Template Separator\n(You can make a copy of, or modify, this frame)"
        n119 = call <vilib>:"Add State(s) to Queue__jki_lib_state_machine.vi"("State(s) in (\"\")"=w335) -> ("States Out"=w334:string)  [unwired: 14 in]
      }
      frame "Enable States: UDP Open" {
        # "Template Separator\n(You can make a copy of, or modify, this frame)"
        # "Open UDP linking to RIB Box."
        n120 = call "FGV - Initialise.vi"("Enum"=FGV_-_Enum."Get Data", "Error In"=w337) -> ("connection ID"=w336:refnum<k16>, "Error Out"=w338:errorcluster)  [unwired: 10 in, 2 out]
        n121 = Bundle By Name(cluster=w341, "connection ID"=w336) -> (w340:T5)
        n122 = call <vilib>:"Add State(s) to Queue__jki_lib_state_machine.vi"("State(s) in (\"\")"=w343) -> ("States Out"=w342:string)  [unwired: 14 in]
      }
      frame "Enable States: Enable ROV A, ROV B and TMS" {
        w371 = u16 54321 ("port or service name")
        # "Data"
        # "Length"
        # "ID"
        # "Target"
        # "Type"
        # "Pkt ID"
        # "Data"
        # "Length"
        # "ID"
        # "Target"
        # "Type"
        # "Pkt ID"
        # "Data"
        # "Length"
        # "ID"
        # "Target"
        # "Type"
        # "Pkt ID"
        # "Send Enable UPS command to RIB Box"
        # "Template Separator\n(You can make a copy of, or modify, this frame)"
        n123 = Unbundle By Name(w351) -> ("connection ID"=w350:refnum<k16>)
        n124 = Build Array(u8 91 ("element"), u8 1 ("element"), u8 9 ("element"), u8 105 ("element"), u8 1 ("element"), u8 1 ("element")) -> (w381:u8[])
        n125 = Byte Array To String(unsigned byte array=w381) -> (string=w378:string)
        n126 = String To IP(1:"192.168.201.21" ("name")) -> (0:w384:u32)
        n127 = UDP Write(address=w384, port or service name=w371, connection ID=w350, data in=w378, 8:w354, 9:1000 ("timeout ms (25000)")) -> (error out=w344:errorcluster, 3:w348:refnum<k16>)
        n128 = Build Array(u8 91 ("element"), u8 1 ("element"), u8 9 ("element"), u8 106 ("element"), u8 1 ("element"), u8 1 ("element")) -> (w382:u8[])
        n129 = Byte Array To String(unsigned byte array=w382) -> (string=w379:string)
        n130 = UDP Write(address=w384, port or service name=w371, connection ID=w348, data in=w379, 8:w344, 9:1000 ("timeout ms (25000)")) -> (error out=w353:errorcluster, 3:w349:refnum<k16>)
        n131 = Build Array(u8 91 ("element"), u8 1 ("element"), u8 9 ("element"), u8 107 ("element"), u8 1 ("element"), u8 1 ("element")) -> (w383:u8[])
        n132 = Byte Array To String(unsigned byte array=w383) -> (string=w380:string)
        n133 = UDP Write(address=w384, port or service name=w371, connection ID=w349, data in=w380, 8:w353, 9:1000 ("timeout ms (25000)")) -> (error out=w347:errorcluster, 3:w352:refnum<k16>)
        n134 = Bundle By Name(cluster=w351, "connection ID"=w352) -> (w385:T5)
        n135 = call <userlib>:"Wait (ms)__ogtk.vi"("error in (no error)"=w347, "milliseconds to wait"=u32 1000) -> ("error out"=w346:errorcluster)  [unwired: 8 in, 1 out]
        n136 = call <vilib>:"Add State(s) to Queue__jki_lib_state_machine.vi"("State(s) in (\"\")"=w387) -> ("States Out"=w386:string)  [unwired: 14 in]
      }
      frame "Enable States: Set Command" {
        # "RIB Box IP"
        # "Data"
        # "Length"
        # "ID"
        # "Target"
        # "Type"
        # "Pkt ID"
        # "SET"
        # "Template Separator\n(You can make a copy of, or modify, this frame)"
        n137 = Unbundle By Name(w405) -> ("connection ID"=w392:refnum<k16>)
        n138 = Build Array(u8 91 ("element"), u8 1 ("element"), u8 9 ("element"), u8 108 ("element"), u8 0 ("element")) -> (w403:u8[])
        n139 = Byte Array To String(unsigned byte array=w403) -> (string=w404:string)
        n140 = String To IP(1:"192.168.201.21" ("name")) -> (0:w396:u32)
        n141 = UDP Write(address=w396, port or service name=u16 54321, connection ID=w392, data in=w404, 8:w394, 9:1000 ("timeout ms (25000)")) -> (error out=w390:errorcluster, 3:w393:refnum<k16>)
        n142 = Bundle By Name(cluster=w405, "connection ID"=w393) -> (w406:T5)
        n143 = call <userlib>:"Wait (ms)__ogtk.vi"("error in (no error)"=w390, "milliseconds to wait"=u32 1000) -> ("error out"=w389:errorcluster)  [unwired: 8 in, 1 out]
        n144 = call <vilib>:"Add State(s) to Queue__jki_lib_state_machine.vi"("State(s) in (\"\")"=w408) -> ("States Out"=w407:string)  [unwired: 14 in]
      }
      frame "Enable States: Start Timer (ROV A)" {
        # "Start 10 second timer"
        # "Template Separator\n(You can make a copy of, or modify, this frame)"
        n145 = call "Timer.vi"("error in (no error)"=w414, "Enum"=T4."Start Timer") -> ("error out"=w413:errorcluster)  [unwired: 6 in, 3 out]
        n146 = property on="Timeout (Read States)" class="Slide (strict)"(error in=w413, "Value"=0.0 ("Horizontal Pointer Slide"), "Scale.Maximum"=15.0 ("Target Time"), "Scale.Minimum"=0.0 ("Scale.Range:Minimum")) -> (error out=w409:errorcluster)  [unwired: 1 in, 1 out]
        n147 = call <vilib>:"Add State(s) to Queue__jki_lib_state_machine.vi"("State(s) in (\"\")"=w418) -> ("States Out"=w417:string)  [unwired: 14 in]
      }
      frame "Enable States: Read ROV A State" {
        # "Read UDP if equal to F0 test complete if not check if timer has elapsed."
        # "#56 = didnt read before the timeout"
        # "Template Separator\n(You can make a copy of, or modify, this frame)"
        n148 = Unbundle By Name(w428) -> ("connection ID"=w438:refnum<k16>)
        n149 = UDP Read(connection ID=w438, timeout ms (25000)=1, 8:w425) -> (data out=w432:string, error out=w431:errorcluster, 3:w429:refnum<k16>)  [unwired: 1 in, 2 out]
        n150 = String Subset(string=w432, offset (0)=15 ("offset (0) 2"), length (rest)=1 ("length (rest) 2")) -> (substring=w434:string)
        n151 = String To Byte Array(string=w434) -> (unsigned byte array=w437:u8[])
        n152 = Number To Hexadecimal String(2:w437) -> (0:w436:string[])  [unwired: 1 in]
        n153 = Index Array(array=w436, index=0) -> (element=w419:string)
        n154 = Equal?(x=w419, y="C") -> (x = y?=w420:bool)
        "ROV A Enabled" <- w420
        n155 = call <vilib>:"Clear Errors.vi"("error in (no error)"=w431, "specific error code to clear (0: all)"=56) -> ("error out"=w426:errorcluster)  [unwired: 4 in, 1 out]
        n156 = Bundle By Name(cluster=w428, "connection ID"=w429, "Read ROV A"=w419) -> (w427:T5)
        n157 = call-poly <vilib>:"Select State(s)__jki_lib_state_machine.vi"("State(s) if True (\"\")"="Macro: Test 2" ("State(s) if True (\"\")"), "Select"=w420, "State(s) if False (\"\")"="Enable States: Elapsed Timer (ROV A)" ("State(s) if False (\"\")")) -> ("States Out"=w421:string)  [unwired: 12 in]
        n158 = call <vilib>:"Add State(s) to Queue__jki_lib_state_machine.vi"("State(s) in Front (\"\")"=w421, "State(s) in (\"\")"=w442) -> ("States Out"=w441:string)  [unwired: 13 in]
      }
      frame "Enable States: Elapsed Timer (ROV A)" {
        # "check if timer elased - if TRUE end test if FALSE read again."
        # "Template Separator\n(You can make a copy of, or modify, this frame)"
        # "Check to see if the timer has elpased."
        n159 = call "Timer.vi"("error in (no error)"=w450, "Target Time"=15.0, "Enum"=T4."Get Time") -> ("error out"=w449:errorcluster, "Time Elapsed?"=w446:bool, "Elapsed Time"=→"Timeout (Read States)":dbl)  [unwired: 5 in, 1 out]
        n160 = call-poly <vilib>:"Select State(s)__jki_lib_state_machine.vi"("State(s) if True (\"\")"="Macro: Test 2" ("State(s) if True (\"\")"), "Select"=w446, "State(s) if False (\"\")"="Enable States: Read ROV A State" ("State(s) if False (\"\")")) -> ("States Out"=w445:string)  [unwired: 12 in]
        n161 = call <vilib>:"Add State(s) to Queue__jki_lib_state_machine.vi"("State(s) in Front (\"\")"=w445, "State(s) in (\"\")"=w454) -> ("States Out"=w453:string)  [unwired: 13 in]
      }
      frame "Enable States: Start Timer (ROV B)" {
        # "Start 10 second timer"
        # "Template Separator\n(You can make a copy of, or modify, this frame)"
        n162 = call "Timer.vi"("error in (no error)"=w460, "Enum"=T4."Start Timer") -> ("error out"=w459:errorcluster)  [unwired: 6 in, 3 out]
        n163 = property on="Timeout (Read States) 2" class="Slide (strict)"(error in=w459, "Value"=0.0 ("Horizontal Pointer Slide"), "Scale.Maximum"=10.0 ("Target Time"), "Scale.Minimum"=0.0 ("Scale.Range:Minimum")) -> (error out=w455:errorcluster)  [unwired: 1 in, 1 out]
        n164 = call <vilib>:"Add State(s) to Queue__jki_lib_state_machine.vi"("State(s) in (\"\")"=w464) -> ("States Out"=w463:string)  [unwired: 14 in]
      }
      frame "Enable States: Read ROV B State" {
        # "Read UDP if equal to F0 test complete if not check if timer has elapsed."
        # "#56 = didnt read before the timeout"
        # "Template Separator\n(You can make a copy of, or modify, this frame)"
        n165 = Unbundle By Name(w471) -> ("connection ID"=w484:refnum<k16>)
        n166 = UDP Read(connection ID=w484, timeout ms (25000)=1, 8:w466) -> (data out=w478:string, error out=w477:errorcluster, 3:w468:refnum<k16>)  [unwired: 1 in, 2 out]
        n167 = String Subset(string=w478, offset (0)=17 ("offset (0) 2"), length (rest)=1 ("length (rest) 2")) -> (substring=w480:string)
        n168 = String To Byte Array(string=w480) -> (unsigned byte array=w483:u8[])
        n169 = Number To Hexadecimal String(2:w483) -> (0:w482:string[])  [unwired: 1 in]
        n170 = Index Array(array=w482, index=0) -> (element=w472:string)
        n171 = Equal?(x=w472, y="F") -> (x = y?=w465:bool)
        "ROV B Enabled" <- w465
        n172 = call <vilib>:"Clear Errors.vi"("error in (no error)"=w477, "specific error code to clear (0: all)"=56) -> ("error out"=w467:errorcluster)  [unwired: 4 in, 1 out]
        n173 = Bundle By Name(cluster=w471, "connection ID"=w468, "Read ROV B"=w472) -> (w470:T5)
        n174 = call-poly <vilib>:"Select State(s)__jki_lib_state_machine.vi"("State(s) if True (\"\")"="Macro: Test 3" ("State(s) if True (\"\")"), "Select"=w465, "State(s) if False (\"\")"="Enable States: Elapsed Timer (ROV B)" ("State(s) if False (\"\")")) -> ("States Out"=w469:string)  [unwired: 12 in]
        n175 = call <vilib>:"Add State(s) to Queue__jki_lib_state_machine.vi"("State(s) in Front (\"\")"=w469, "State(s) in (\"\")"=w488) -> ("States Out"=w487:string)  [unwired: 13 in]
      }
      frame "Enable States: Elapsed Timer (ROV B)" {
        # "check if timer elased - if TRUE end test if FALSE read again."
        # "Template Separator\n(You can make a copy of, or modify, this frame)"
        # "Check to see if the timer has elpased."
        n176 = call "Timer.vi"("error in (no error)"=w496, "Target Time"=10.0, "Enum"=T4."Get Time") -> ("error out"=w495:errorcluster, "Time Elapsed?"=w492:bool, "Elapsed Time"=→"Timeout (Read States) 2":dbl)  [unwired: 5 in, 1 out]
        n177 = call-poly <vilib>:"Select State(s)__jki_lib_state_machine.vi"("State(s) if True (\"\")"="Macro: Test 3" ("State(s) if True (\"\")"), "Select"=w492, "State(s) if False (\"\")"="Enable States: Read ROV B State" ("State(s) if False (\"\")")) -> ("States Out"=w491:string)  [unwired: 12 in]
        n178 = call <vilib>:"Add State(s) to Queue__jki_lib_state_machine.vi"("State(s) in Front (\"\")"=w491, "State(s) in (\"\")"=w500) -> ("States Out"=w499:string)  [unwired: 13 in]
      }
      frame "Enable States: Start Timer (TMS)" {
        # "Start 10 second timer"
        # "Template Separator\n(You can make a copy of, or modify, this frame)"
        n179 = call "Timer.vi"("error in (no error)"=w506, "Enum"=T4."Start Timer") -> ("error out"=w505:errorcluster)  [unwired: 6 in, 3 out]
        n180 = property on="Timeout (Read States) 3" class="Slide (strict)"(error in=w505, "Value"=0.0 ("Horizontal Pointer Slide"), "Scale.Maximum"=10.0 ("Target Time"), "Scale.Minimum"=0.0 ("Scale.Range:Minimum")) -> (error out=w501:errorcluster)  [unwired: 1 in, 1 out]
        n181 = call <vilib>:"Add State(s) to Queue__jki_lib_state_machine.vi"("State(s) in (\"\")"=w510) -> ("States Out"=w509:string)  [unwired: 14 in]
      }
      frame "Enable States: Read TMS State" {
        # "Read UDP if equal to F0 test complete if not check if timer has elapsed."
        # "#56 = didnt read before the timeout"
        # "Template Separator\n(You can make a copy of, or modify, this frame)"
        n182 = Unbundle By Name(w517) -> ("connection ID"=w530:refnum<k16>)
        n183 = UDP Read(connection ID=w530, timeout ms (25000)=1, 8:w512) -> (data out=w524:string, error out=w523:errorcluster, 3:w514:refnum<k16>)  [unwired: 1 in, 2 out]
        n184 = String Subset(string=w524, offset (0)=19 ("offset (0) 2"), length (rest)=1 ("length (rest) 2")) -> (substring=w526:string)
        n185 = String To Byte Array(string=w526) -> (unsigned byte array=w529:u8[])
        n186 = Number To Hexadecimal String(2:w529) -> (0:w528:string[])  [unwired: 1 in]
        n187 = Index Array(array=w528, index=0) -> (element=w518:string)
        n188 = Equal?(x=w518, y="12") -> (x = y?=w511:bool)
        "TMS Enabled" <- w511
        n189 = call <vilib>:"Clear Errors.vi"("error in (no error)"=w523, "specific error code to clear (0: all)"=56) -> ("error out"=w513:errorcluster)  [unwired: 4 in, 1 out]
        n190 = Bundle By Name(cluster=w517, "connection ID"=w514, "Read TMS"=w518) -> (w516:T5)
        n191 = call-poly <vilib>:"Select State(s)__jki_lib_state_machine.vi"("State(s) if True (\"\")"="Macro: Limits" ("State(s) if True (\"\")"), "Select"=w511, "State(s) if False (\"\")"="Enable States: Elapsed Timer (TMS)" ("State(s) if False (\"\")")) -> ("States Out"=w515:string)  [unwired: 12 in]
        n192 = call <vilib>:"Add State(s) to Queue__jki_lib_state_machine.vi"("State(s) in Front (\"\")"=w515, "State(s) in (\"\")"=w534) -> ("States Out"=w533:string)  [unwired: 13 in]
      }
      frame "Enable States: Elapsed Timer (TMS)" {
        # "check if timer elased - if TRUE end test if FALSE read again."
        # "Template Separator\n(You can make a copy of, or modify, this frame)"
        # "Check to see if the timer has elpased."
        n193 = call "Timer.vi"("error in (no error)"=w542, "Target Time"=10.0, "Enum"=T4."Get Time") -> ("error out"=w541:errorcluster, "Time Elapsed?"=w538:bool, "Elapsed Time"=→"Timeout (Read States) 3":dbl)  [unwired: 5 in, 1 out]
        n194 = call-poly <vilib>:"Select State(s)__jki_lib_state_machine.vi"("State(s) if True (\"\")"="Macro: Limits" ("State(s) if True (\"\")"), "Select"=w538, "State(s) if False (\"\")"="Enable States: Read TMS State" ("State(s) if False (\"\")")) -> ("States Out"=w537:string)  [unwired: 12 in]
        n195 = call <vilib>:"Add State(s) to Queue__jki_lib_state_machine.vi"("State(s) in Front (\"\")"=w537, "State(s) in (\"\")"=w546) -> ("States Out"=w545:string)  [unwired: 13 in]
      }
    }
    n196 = Wait (ms)(milliseconds to wait=u32 2) -> ()  [unwired: 1 out]
  }
  "error out" <- w1
